vi "Generate Data.vi"(0 "Datapoints":i32) -> (1 "Index":i32[](array[numeric]), 2 "Time":dbl[unit][](array[numeric]), 3 "Voltage":dbl[unit][](array[numeric]), 4 "Current":dbl[unit][](array[numeric]))   [LabVIEW 2018]
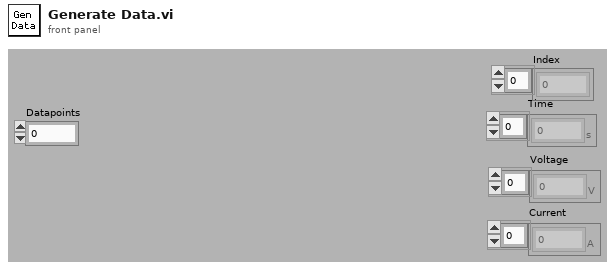
[diagram p1: front panel]
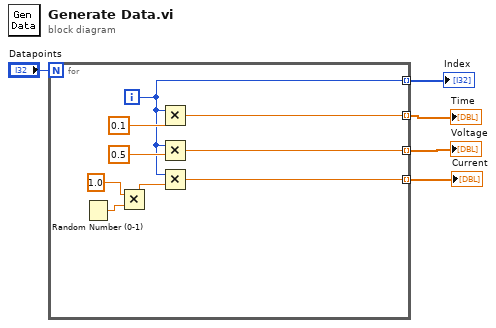
[diagram p0: block diagram]
diagram:
  n1 = for {
    N: "Datapoints" -> [_]
    tunnel: [w9] -> w2 mode=indexing
    tunnel: [w8] -> w3 mode=indexing
    tunnel: [w7] -> w4 mode=indexing
    tunnel: [w6] -> w1 mode=indexing
    i -> [w6]
    n2 = Random Number (0-1)() -> (number: 0 to 1=w13:dbl)
    n3 = Multiply(x=dbl[unit] 1.0 ("y"), y=w13) -> (x*y=w11:dbl[unit])
    n4 = Multiply(x=w6, y=dbl[unit] 0.1) -> (x*y=w7:dbl[unit])
    n5 = Multiply(x=w6, y=dbl[unit] 0.5) -> (x*y=w8:dbl[unit])
    n6 = Multiply(x=w6, y=w11) -> (x*y=w9:dbl[unit])
  }
  "Time" <- w4
  "Voltage" <- w3
  "Current" <- w2
  "Index" <- w1
